vi "Continuous File Read.vi"(11 "file path":path) -> (0 "error out":errorcluster)   [LabVIEW 2018]
doc: "Attempts to open (read-only) and continuously read a text file and display the output to the front panel. Useful for streaming stdout that's being piped into a file."
panel:
  in  "stop":bool
  out "text":string
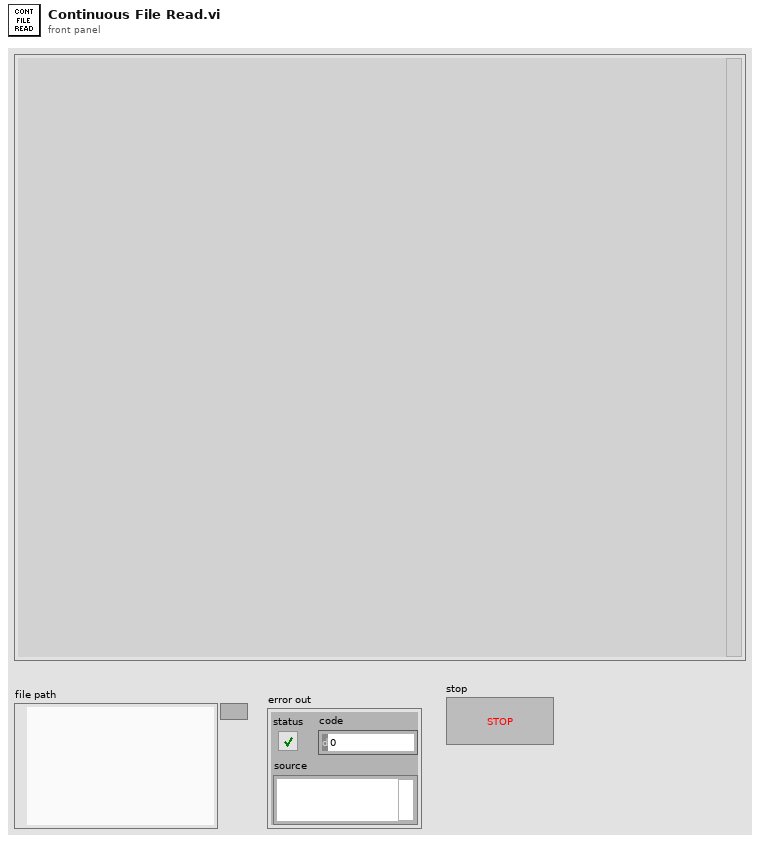
[diagram p1: front panel]
types:
  T1 = enum32{"Invalid", "Standard", "Closed", "Hidden", "Minimized", "Maximized"}
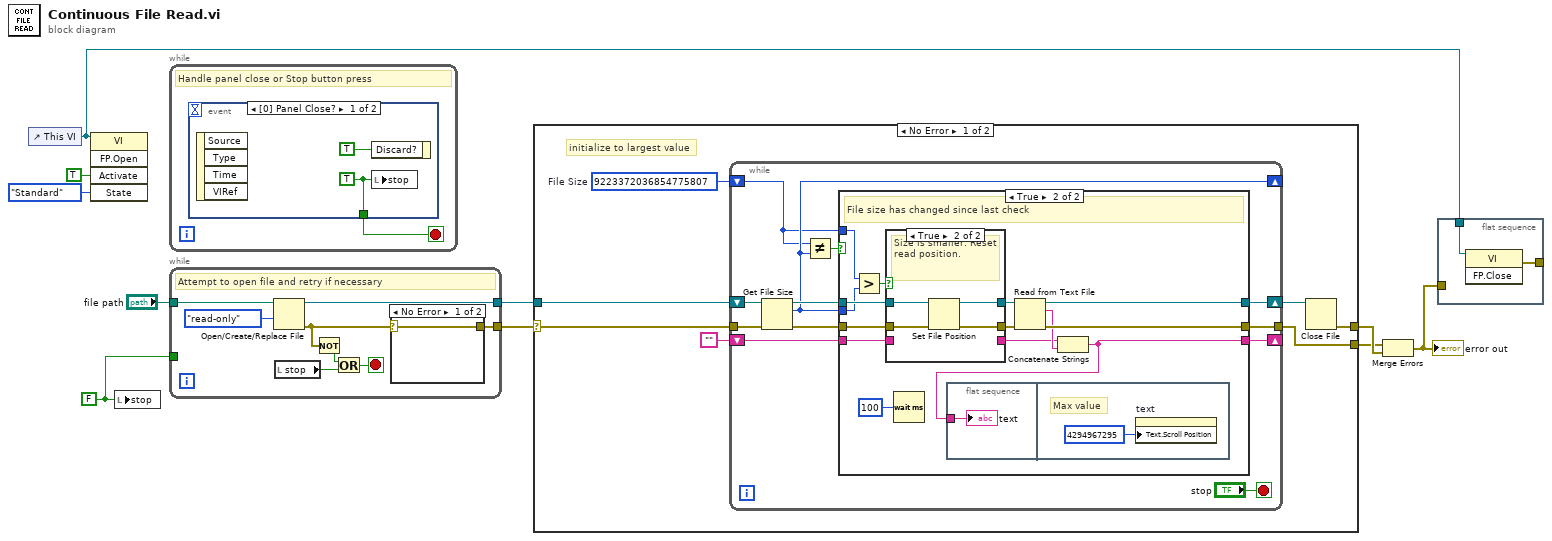
[diagram p0: block diagram]
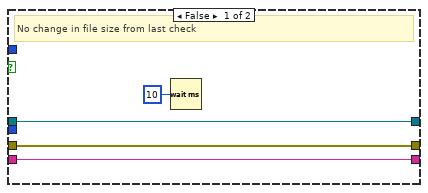
[diagram p2: hidden frame]
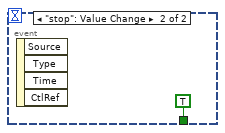
[diagram p5: hidden frame]
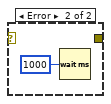
[diagram p6: hidden frame]
diagram:
  w6 = FALSE ("stop")
  n1 = control-ref of="This VI"() -> (w1:refnum<vi>)
  n2 = invoke class="VI" method="FP.Open"(reference=w1, "Activate"=TRUE ("Activate?"), "State"=T1."Standard") -> ()  [unwired: 2 in, 5 out]
  n3 = local write "stop"(w6) -> ()
  n4 = while {
    stop <- w11 stop-if-true
    # "Handle panel close or Stop button press"
    n5 = event shown="[0] Panel Close?" {
      selector: _ -> [_ _]
      dyn-events: _ -> [_ _]
      timeout: _ -> [_ _]
      tunnel: [w12 TRUE] -> w11
      event Panel Close? {
        w12 = TRUE
        n6 = event-data() -> ()  [unwired: 1 in, 4 out]
        n7 = event-data("Discard?"=TRUE) -> ()  [unwired: 1 in, 1 out]
        n8 = local write "stop"(w12) -> ()
      }
      event "stop": Value Change {
        n9 = event-data() -> ()  [unwired: 1 in, 4 out]
      }
    }
  }
  n10 = while {
    tunnel: [w18] -> w10
    tunnel: [w21] -> w9
    tunnel: "file path" -> [w20]
    tunnel: w6 -> [_]
    stop <- w16 stop-if-true
    # "Attempt to open file and retry if necessary"
    n11 = Open/Create/Replace File(file path (use dialog)=w20, access (0:read/write)=enum16{"read/write", "read-only", "write-only"}."read-only") -> (refnum out=w21:refnum<file>, error out=w19:errorcluster)  [unwired: 4 in, 1 out]
    n12 = local read "stop"() -> (w15:bool)
    n13 = Not(x=w19) -> (.not. x?=w17:bool)
    n14 = Or(x=w17, y=w15) -> (x .or. y?=w16:bool)
    n15 = case shown="No Error" w19 {
      selector: w19 -> [w23 _]
      tunnel: [w23 _] -> w18
      frame No Error {
      }
      frame Error {
        n16 = Wait (ms)(milliseconds to wait=u32 1000) -> ()  [unwired: 1 out]
      }
    }
  }
  n17 = case shown="No Error" w10 {
    selector: w10 -> [w31 w71]
    tunnel: w9 -> [w30 _]
    tunnel: [w25 w71] -> w8
    tunnel: [w26 w71] -> w7
    frame No Error {
      w28 = i64 9223372036854775807  # File Size
      # "initialize to largest value"
      n18 = while {
        tunnel: w31 -> [w32]
        tunnel: [w42] -> w26
        shift-right: [w40] -> _
        shift-left: "" -> [w36]
        shift-right: [w35] -> _
        shift-left: w28 -> [w34]
        shift-right: [w41] -> w27
        shift-left: w30 -> [w39]
        stop <- "stop" stop-if-true
        n19 = Get File Size(file=w39, error in=w32) -> (refnum out=w37:refnum<file>, size (in bytes)=w35:i64, 0:w38:errorcluster)
        n20 = Not Equal?(x=w34, y=w35) -> (x != y?=w33:bool)
        n21 = case shown="True" w33 {
          tunnel: [w45 w60] -> w42
          tunnel: [w46 w59] -> w41
          tunnel: [w47 w48] -> w40
          tunnel: w38 -> [w45 w57]
          tunnel: w37 -> [w46 w56]
          tunnel: w34 -> [_ w55]
          tunnel: w35 -> [_ w52]
          tunnel: w36 -> [w47 w51]
          frame False {
            # "No change in file size from last check"
            n22 = Wait (ms)(milliseconds to wait=u32 10) -> ()  [unwired: 1 out]
          }
          frame True {
            # "File size has changed since last check"
            n23 = Greater?(x=w55, y=w52) -> (0:w54:bool)
            n24 = case shown="True" w54 {
              tunnel: w57 -> [w64 w70]
              tunnel: w56 -> [w66 w69]
              tunnel: [w66 w68] -> w53
              tunnel: w51 -> [w65 _]
              tunnel: [w65 _] -> w49
              tunnel: [w64 w67] -> w50
              frame False {
                # "File size is >= previous. Read from current position."
              }
              frame True {
                # "Size is smaller. Reset read position."
                n25 = Set File Position(refnum=w69, error in=w70) -> (refnum out=w68:refnum<file>, error out=w67:errorcluster)  [unwired: 2 in]
              }
            }
            n26 = Wait (ms)(milliseconds to wait=u32 100) -> ()  [unwired: 1 out]
            n27 = flat-sequence {
              tunnel: w48 -> [w62]
              frame #0 {
                "text" <- w62
              }
              frame #1 {
                # "Max value"
                n28 = property on="text" class="Str"("Text.Scroll Position"=u32 4294967295) -> ()  [unwired: 2 in, 2 out]
              }
            }
            n29 = Read from Text File(file (use dialog)=w53, error in=w50) -> (refnum out=w59:refnum<file>, text=w58:string, error out=w60:errorcluster)  [unwired: 2 in, 1 out]
            n30 = Concatenate Strings(w49, w58) -> (w48:string)
          }
        }
      }
      n31 = Close File(refnum=w27) -> (error out=w25:errorcluster)  [unwired: 1 in, 1 out]
    }
    frame Error {
    }
  }
  n32 = Merge Errors(w7, w8) -> (w2:errorcluster)
  "error out" <- w2
  n33 = flat-sequence {
    tunnel: w2 -> [_]
    tunnel: w1 -> [w73]
    tunnel: [w72] -> _
    frame #0 {
      n34 = invoke class="VI" method="FP.Close"(reference=w73) -> (error out=w72:errorcluster)  [unwired: 2 in, 2 out]
    }
  }
